vi "GEN40-38-LAN Send Command.vi"(8 "error in (no error)":errorcluster, 9 "Wait for Response?":bool, 10 "Command":string, 11 "VISA resource name":refnum<visa-resource-name>) -> (0 "error out":errorcluster, 2 "Response":string, 3 "VISA resource name out":refnum<visa-resource-name>)   [LabVIEW 2018, in "GEN40-38-LAN.lvlib" / "GEN40-38-LAN.lvclass"]
doc: "This VI is used to send anc command to the Power Supply and also reads the command response, if expected."
uses:
  GEN40-38-LAN.lvclass
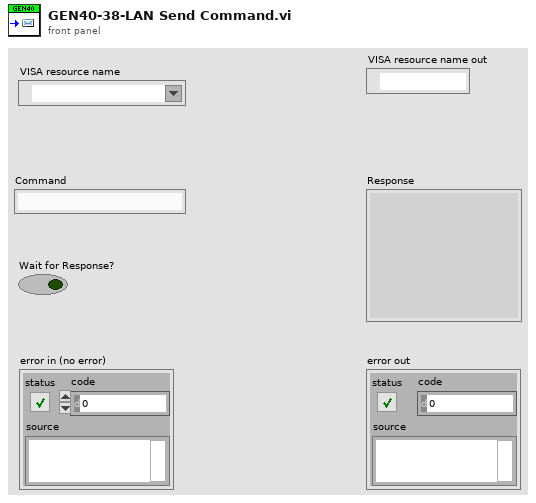
[diagram p1: front panel]
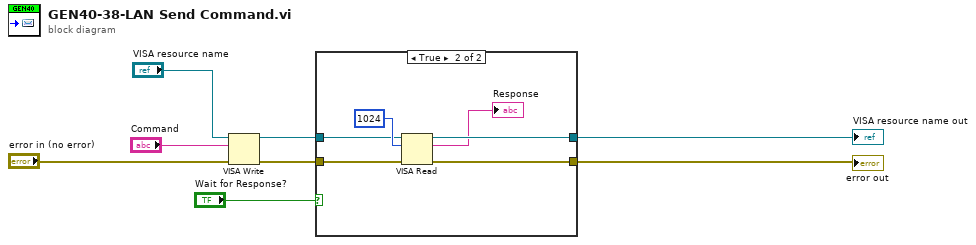
[diagram p0: block diagram]
diagram:
  n1 = VISA Write(VISA resource name="VISA resource name", write buffer="Command", error in (no error)="error in (no error)") -> (VISA resource name out=w8:refnum<visa-resource-name>, error out=w7:errorcluster)  [unwired: 1 out]
  n2 = case shown="True" "Wait for Response?" {
    tunnel: w8 -> [w10 w15]
    tunnel: w7 -> [w9 w14]
    tunnel: [w10 w13] -> w2
    tunnel: [w9 w12] -> w1
    frame False {
    }
    frame True {
      n3 = VISA Read(VISA resource name=w15, byte count=u32 1024, error in (no error)=w14) -> (VISA resource name out=w13:refnum<visa-resource-name>, read buffer=→"Response":string, error out=w12:errorcluster)  [unwired: 1 out]
    }
  }
  "VISA resource name out" <- w2
  "error out" <- w1
